vi "set home settings calb.vi"(8 "error in (no error)":errorcluster, 9 "calibration":cluster{"A":dbl, "MicrostepMode":u32}, 10 "home_settings_calb":T1, 11 "id":i32) -> (0 "error out":errorcluster, 3 "function return":i32)   [LabVIEW 2012, in "libximc.lvlib"]
doc: "result_t XIMC_API set_home_settings_calb (device_t id, const home_settings_calb_t* home_settings_calb, const calibration_t* calibration);"
uses:
  libximc.lvlib
  libximc.dll
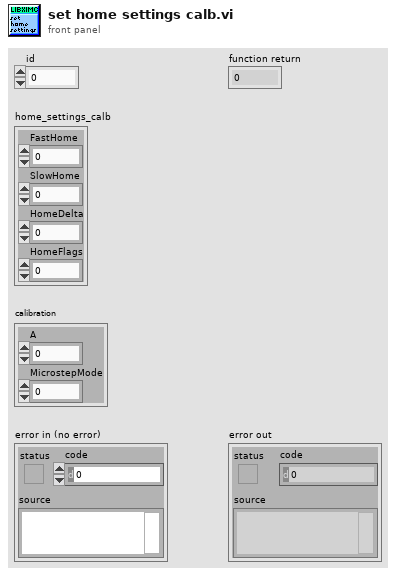
[diagram p1: front panel]
types:
  T1 = cluster{"FastHome":sgl, "SlowHome":sgl, "HomeDelta":sgl, "HomeFlags":u32}
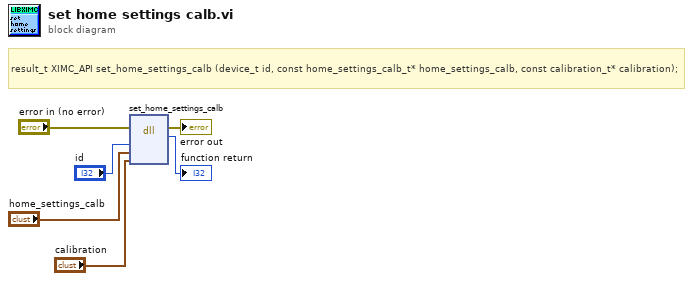
[diagram p0: block diagram]
diagram:
  # "result_t XIMC_API set_home_settings_calb (device_t id, const home_settings_calb_t* home_settings_calb, const calibration_t* calibration);"
  n1 = dll-call lib="E:/labview-2.12.1-Labview_12.0/ximcLVx32/libximc.*" fn="set_home_settings_calb"(error in="error in (no error)", "id"="id", "home_settings_calb"="home_settings_calb", "calibration"="calibration") -> (error out=→"error out":errorcluster, →"function return":i32)  [unwired: 5 in, 1 out]
